vi "sfrgergerger.vi"() -> ()   [LabVIEW 2016]
uses:
  <vilib>/CANopenLib/CANOPEN.llb/CANopen SDO Create.vi
  Get Error.vi
panel:
  out "Error code":u16
  in  "Motor":u8(ring) items=["Right", "Left"]
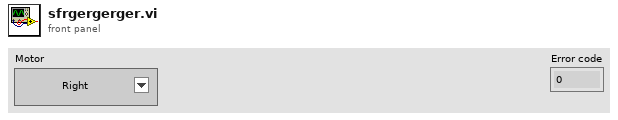
[diagram p1: front panel]
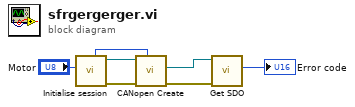
[diagram p0: block diagram]
diagram:
  n1 = call "Initialise session.vi"("Motor"="Motor") -> ("error out"=w6:errorcluster, "interface object out"=w7:refnum<k20>, "Used Node ID"=w1:u8)  [unwired: 8 in]
  n2 = call-poly <vilib>:"CANopen Create.vi"("node-ID"=w1, "error in (no error)"=w6, "interface object in"=w7) -> ("error out"=w3:errorcluster, "SDO object out"=w4:refnum<k20>)  [unwired: 6 in, 1 out]
  n3 = call-poly "Get SDO.vi"("error in (no error)"=w3, "SDO object in"=w4) -> ("Error code"=→"Error code":u16)  [unwired: 5 in, 4 out]
